vi "Open Trace File.vi"(4 "Data Type":T2(ring)=enum."float32", 6 "File Type ID":string="WFM", 8 "Error In":errorcluster, 11 "File Path":path) -> (0 "Error Out":errorcluster, 3 "File Refnum Out":refnum<file>)   [LabVIEW 2015]
uses:
  Processing/Trace (dbl).ctl
panel:
  in  "Trace":T1
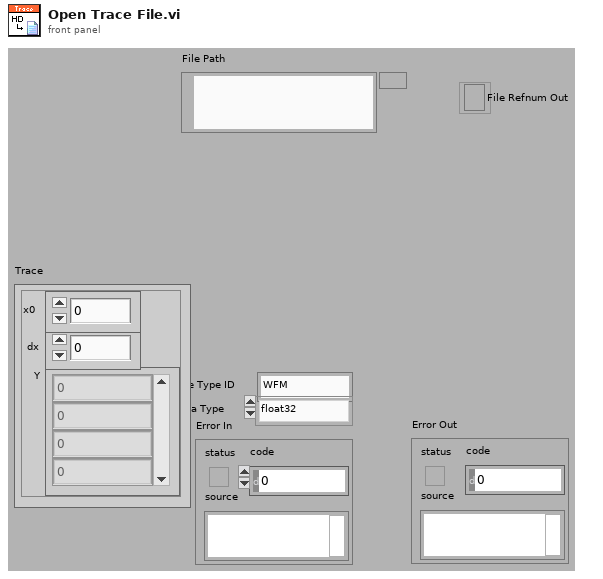
[diagram p1: front panel]
types:
  T1 = typedef "Trace (dbl).ctl" = cluster{"x0 ":dbl, "dx":dbl, "Y":dbl[]}
  T2 = enum16{"int8", "int16", "int32", "uint8", "uint16", "uint32", "float32", "float64"}
  T3 = enum16{"open", "replace", "create", "open or create", "replace or create", "replace or create with confirmation"}
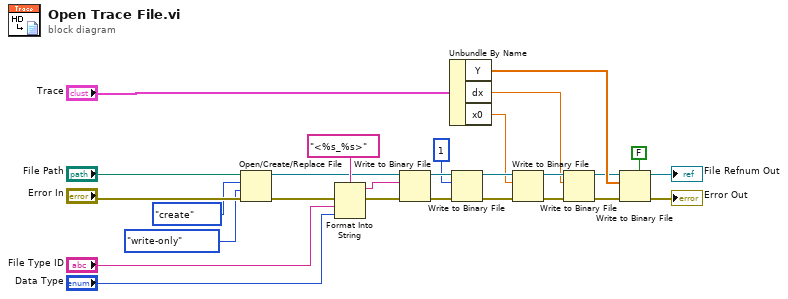
[diagram p0: block diagram]
diagram:
  n1 = Open/Create/Replace File(file path (use dialog)="File Path", error in="Error In", operation (0:open)=T3."create", access (0:read/write)=enum16{"read/write", "read-only", "write-only"}."write-only") -> (refnum out=w8:refnum<file>, error out=w9:errorcluster)  [unwired: 2 in, 1 out]
  n2 = Format Into String(format string="<%s_%s>", error in=w9, "File Type ID", "Data Type") -> (resulting string=w12:string, error out=w19:errorcluster)  [unwired: 1 in]
  n3 = Write to Binary File(file (use dialog)=w8, data=w12, error in=w19) -> (refnum out=w14:refnum<file>, error out=w13:errorcluster)  [unwired: 3 in, 1 out]
  n4 = Unbundle By Name("Trace") -> ("Y"=w5:dbl[], "dx"=w1:dbl, "x0"=w2:dbl)
  n5 = Write to Binary File(file (use dialog)=w14, data=1 ("No. of Channels"), error in=w13) -> (refnum out=w15:refnum<file>, error out=w17:errorcluster)  [unwired: 3 in, 1 out]
  n6 = Write to Binary File(file (use dialog)=w15, data=w2, error in=w17) -> (refnum out=w16:refnum<file>, error out=w18:errorcluster)  [unwired: 3 in, 1 out]
  n7 = Write to Binary File(file (use dialog)=w16, data=w1, error in=w18) -> (refnum out=w4:refnum<file>, error out=w3:errorcluster)  [unwired: 3 in, 1 out]
  n8 = Write to Binary File(file (use dialog)=w4, data=w5, error in=w3, 5:FALSE ("prepend array or string size? (T)")) -> (refnum out=→"File Refnum Out":refnum<file>, error out=→"Error Out":errorcluster)  [unwired: 2 in, 1 out]
